vi "Mercury Query.vi"(8 "Error In":errorcluster, 9 "byte count":i32=4096 caption="byte count (4096)", 10 "Command":string, 11 "VISA resource name":refnum<visa-resource-name>) -> (0 "Error Out":errorcluster, 2 "Response":string, 3 "VISA resource name out":refnum<visa-resource-name>)   [LabVIEW 2015]
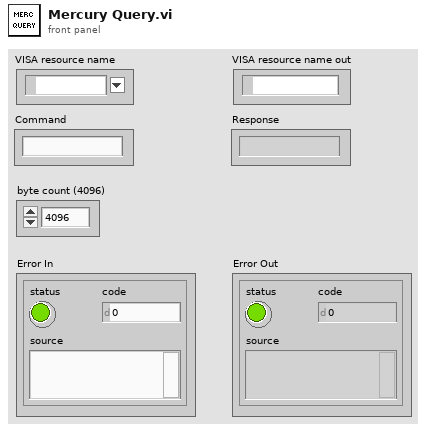
[diagram p1: front panel]
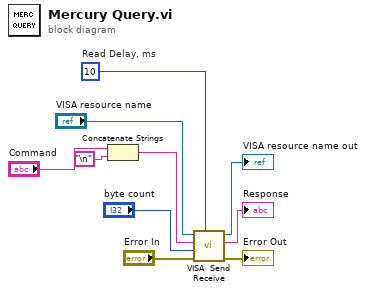
[diagram p0: block diagram]
diagram:
  w9 = u32 10  # Read Delay, ms
  n1 = Concatenate Strings("Command", "\n") -> (w2:string)
  n2 = call "VISA  Send Receive.vi"("Read Delay, ms"=w9, "error in (no error)"="Error In", "Receive count"="byte count", "data string in"=w2, "VISA Resource Name"="VISA resource name") -> ("error out"=→"Error Out":errorcluster, "data string out"=→"Response":string, "VISA Resource Name Out"=→"VISA resource name out":refnum<visa-resource-name>)  [unwired: 4 in]
